vi "LogFileGlobals.vi"() -> ()   [LabVIEW 2017]
panel:
  in  "FileRef":refnum<file>
  out "FileSize":u32
  in  "file path":path
  in  "NoOfEntries":u32
  in  "Chars/Entry":u32
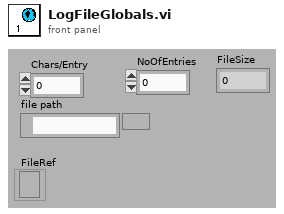
[diagram p1: front panel]
diagram:
